vi "Version 1_Read Register.vi"(7 "Address (A)":string="A", 8 "error in":errorcluster, 11 "VISA Session In":refnum<visa-resource-name>="Alicat") -> (0 "error out":errorcluster, 1 "Register Value (Legacy)":i16 format="%.0x", 2 "Register Value (U32)":i32 format="%.0x", 3 "VISA Session Out":refnum<visa-resource-name>)   [LabVIEW 2015]
panel:
  in  "Register address":i16
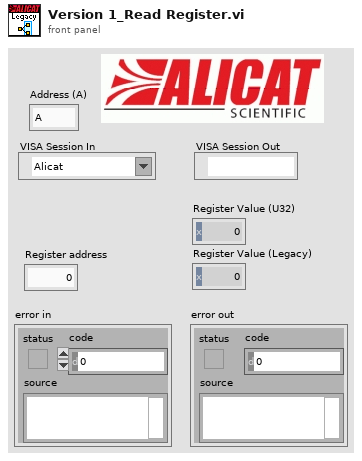
[diagram p1: front panel]
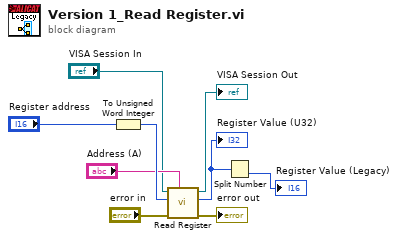
[diagram p0: block diagram]
diagram:
  n1 = To Unsigned Word Integer(number="Register address") -> (unsigned 16bit integer=w8:u16)
  n2 = call "Read Register.vi"("Unit ID (A)"="Address (A)", "error in"="error in", "Register address"=w8, "VISA Session In"="VISA Session In") -> ("error out"=→"error out":errorcluster, "Register Value (I32)"=w7:i32, "VISA Session Out"=→"VISA Session Out":refnum<visa-resource-name>)  [unwired: 5 in]
  "Register Value (U32)" <- w7
  n3 = Split Number(x=w7) -> (lo(x)=→"Register Value (Legacy)":u16)  [unwired: 1 out]
